vi "Configure Surge-Drop Mode.vi"(0 "VISA resource name":refnum<visa-resource-name>, 5 "Enable Surge Drop (F:Disable)":bool, 11 "error in (no error)":errorcluster) -> (4 "VISA resource name out":refnum<visa-resource-name>, 15 "error out":errorcluster)   [LabVIEW 2016, in "APT 300XAC Series.lvlib"]
doc: "Enables or Disables the <B>Surge Drop</B> in the power source instrument. \n\nThe surge/drop parameter configures or trigger surges or drops in the voltage output when in either the program or manual mode.\n\nNote :\nProgram Mode : Step Parameter (Can be configured in every step individually).\nManual Mode : System Parameter ( Change in mode affect all steps and memory)\nDC Mode : Not Supported"
uses:
  APT 300XAC Series.lvlib
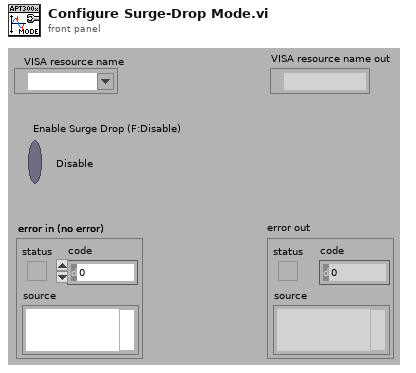
[diagram p1: front panel]
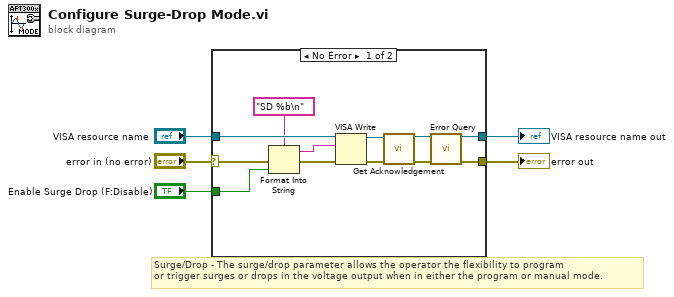
[diagram p0: block diagram]
diagram:
  # "Surge/Drop - The surge/drop parameter allows the operator the flexibility to program \nor trigger surges or drops in the voltage output when in either the program or manual mode."
  n1 = case shown="No Error" "error in (no error)" {
    selector: "error in (no error)" -> [w12 w19]
    tunnel: "VISA resource name" -> [w17 w18]
    tunnel: [w14 w18] -> w4
    tunnel: [w13 w19] -> w3
    tunnel: "Enable Surge Drop (F:Disable)" -> [w10 _]
    frame No Error {
      n2 = Format Into String(format string="SD %b\n" ("Command"), error in=w12, w10) -> (resulting string=w16:string, error out=w11:errorcluster)  [unwired: 1 in]
      n3 = VISA Write(VISA resource name=w17, write buffer=w16, error in (no error)=w11) -> (VISA resource name out=w6:refnum<visa-resource-name>, error out=w7:errorcluster)  [unwired: 1 out]
      n4 = call "Get Acknowledgement.vi"("VISA resource name"=w6, "error in (no error)"=w7) -> ("VISA resource name out"=w8:refnum<visa-resource-name>, "error out"=w9:errorcluster)  [unwired: 12 in]
      n5 = call "Error Query.vi"("VISA resource name"=w8, "error in (no error)"=w9) -> ("VISA resource name out"=w14:refnum<visa-resource-name>, "error out"=w13:errorcluster)  [unwired: 10 in, 2 out]
    }
    frame Error {
    }
  }
  "error out" <- w3
  "VISA resource name out" <- w4
